vi "Thread@SubThreadStart__Parameter.vi"(1 "ParamterIn":string) -> (0 "ParamterOut":string)   [LabVIEW 2020]
panel:
  in  "Logic":string(combo)
  in  "SubName":string(combo)
  in  "Confirm":bool
  # "Thread@SubThreadStart $SubName(,$Logic)\nIf $SubName has \"&\" at end, it's \"Background Process\" \nIf $SubName has \"&&\" at end, it's \"MultiThread Mode\""
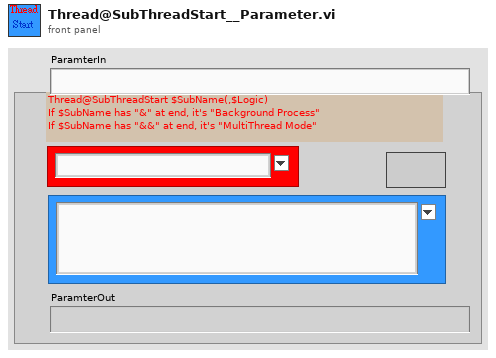
[diagram p1: front panel]
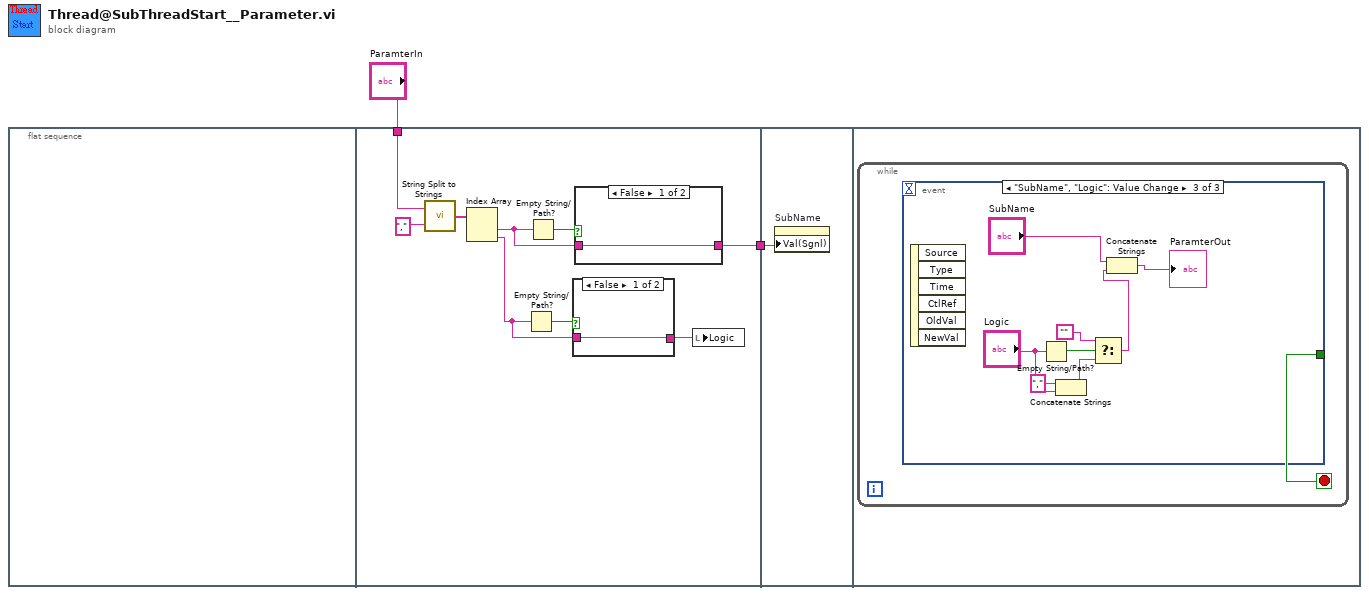
[diagram p0: block diagram]
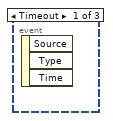
[diagram p4: hidden frame]
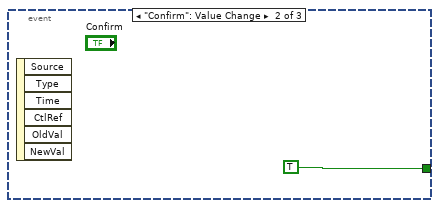
[diagram p5: hidden frame]
diagram:
  n1 = flat-sequence {
    tunnel: "ParamterIn" -> [w9]
    tunnel: [w4] -> w1
    tunnel: w1 -> [w14]
    frame #0 {
    }
    frame #1 {
      n2 = call "String Split to Strings.vi"("search string/char (-)"=",", "String"=w9) -> ("Array"=w11:string[])
      n3 = Index Array(array=w11) -> (element #1=w7:string, element #2=w5:string)  [unwired: 2 in]
      n4 = Empty String/Path?(string/path=w5) -> (empty?=w6:bool)
      n5 = Empty String/Path?(string/path=w7) -> (empty?=w8:bool)
      n6 = case shown="False" w6 {
        tunnel: w5 -> [w12 _]
        tunnel: [w12 _] -> w3
        frame False {
        }
        frame True {
        }
      }
      n7 = case shown="False" w8 {
        tunnel: w7 -> [w13 _]
        tunnel: [w13 _] -> w4
        frame False {
        }
        frame True {
        }
      }
      n8 = local write "Logic"(w3) -> ()
    }
    frame #2 {
      n9 = property on="SubName" class="CmbBox"("Val(Sgnl)"=w14) -> ()  [unwired: 2 in, 2 out]
    }
    frame #3 {
      n10 = while {
        stop <- w15 stop-if-true
        n11 = event shown="[2] \"SubName\", \"Logic\": Value Change" {
          selector: _ -> [_ _ _]
          dyn-events: _ -> [_ _ _]
          timeout: _ -> [_ _ _]
          tunnel: [_ TRUE _] -> w15
          event Timeout {
            n12 = event-data() -> ()  [unwired: 1 in, 3 out]
          }
          event "Confirm": Value Change {
            n13 = event-data() -> ()  [unwired: 1 in, 6 out]
          }
          event "SubName", "Logic": Value Change {
            n14 = event-data() -> ()  [unwired: 1 in, 6 out]
            n15 = Empty String/Path?(string/path="Logic") -> (empty?=w23:bool)
            n16 = Concatenate Strings("," ("string"), "Logic") -> (w21:string)
            n17 = Select(t="", s=w23, f=w21) -> (s? t:f=w18:string)
            n18 = Concatenate Strings("SubName", w18) -> (→"ParamterOut":string)
          }
        }
      }
    }
  }
